vi "Catch.vi"(7 "Action":T1, 8 "error in (no error)":errorcluster) -> (0 "error out":errorcluster)   [LabVIEW 2015]
doc: "Wrapper for catching. It has the following actions:\n-PreCatch: sets the clapper to out, the roller pneumatic to in, actuates the kicker, and spins the roller motor forward.\n-Catch: sets the clapper to in.\n-Stop: deactuates the kicker, turns the roller motor off, and sets the roller pneumatic to middle."
uses:
  CatchAction.ctl
  DoubleSolenoidAction.ctl
  RollerAction.ctl
  SingleSolenoidAction.ctl
  PnuematicMode.ctl
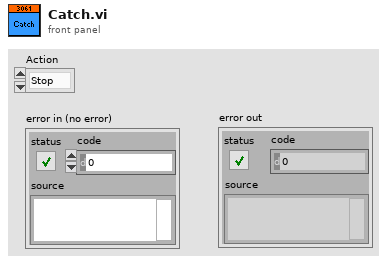
[diagram p1: front panel]
types:
  T1 = typedef "CatchAction.ctl" = enum16{"Stop", "PreCatch", "Catch"}
  T2 = typedef "SingleSolenoidAction.ctl" = enum16{"Init", "SetState", "Disable"}
  T3 = typedef "RollerAction.ctl" = enum16{"Init", "Off", "Forward", "Reverse"}
  T4 = typedef "DoubleSolenoidAction.ctl" = enum16{"Init", "Middle", "In", "Out"}
  T5 = typedef "PnuematicMode.ctl" = enum16{"Init", "SetState", "Disable"}
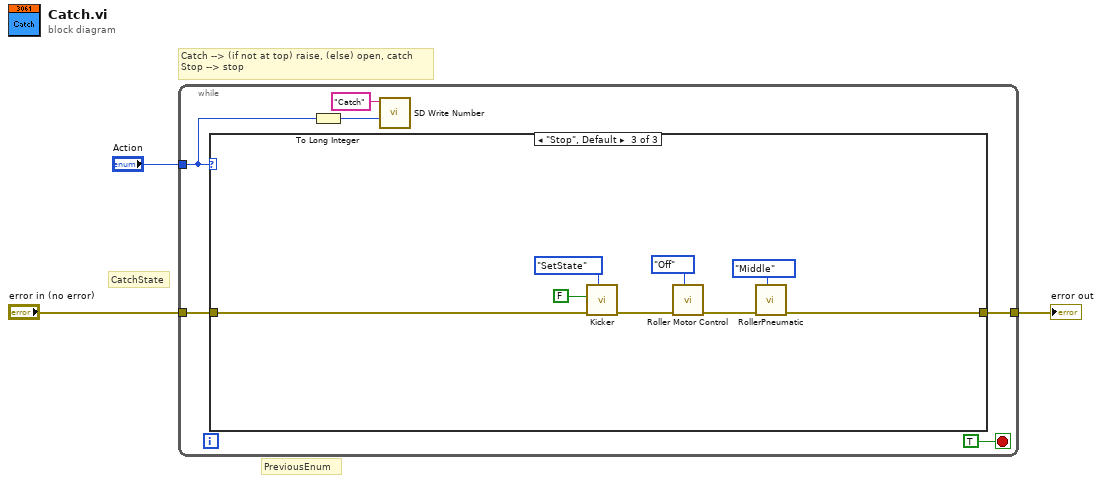
[diagram p0: block diagram]
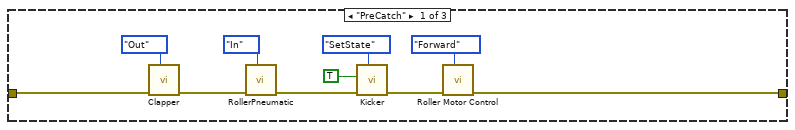
[diagram p2: hidden frame]
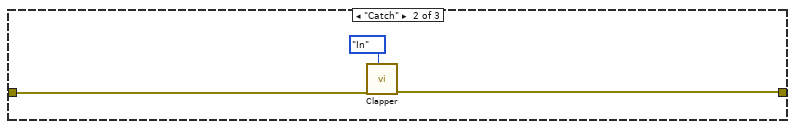
[diagram p3: hidden frame]
diagram:
  # "CatchState"
  # "Catch --> (if not at top) raise, (else) open, catch\nStop --> stop"
  # "PreviousEnum"
  n1 = while {
    tunnel: "error in (no error)" -> [w9]
    tunnel: [w8] -> w2
    tunnel: "Action" -> [w4]
    stop <- TRUE stop-if-true
    n2 = case shown="\"Stop\", Default" w4 {
      tunnel: w9 -> [w14 w21 w26]
      tunnel: [w12 w20 w24] -> w8
      frame "PreCatch" {
        n3 = call "Clapper.vi"("State"=DoubleSolenoidAction."Out", "Error in"=w14) -> ("Error out"=w15:errorcluster)  [unwired: 9 in]
        n4 = call "RollerPneumatic.vi"("State"=DoubleSolenoidAction."In", "Error in"=w15) -> ("Error out"=w16:errorcluster)  [unwired: 9 in]
        n5 = call "Kicker.vi"("Action"=SingleSolenoidAction."SetState", "error in (no error)"=w16, "Actuate?"=TRUE) -> ("error out"=w13:errorcluster)  [unwired: 8 in]
        n6 = call "Roller Motor Control.vi"("Action"=RollerAction."Forward", "Error in"=w13) -> ("Error out"=w12:errorcluster)  [unwired: 9 in]
      }
      frame "Catch" {
        n7 = call "Clapper.vi"("State"=DoubleSolenoidAction."In", "Error in"=w21) -> ("Error out"=w20:errorcluster)  [unwired: 9 in]
      }
      frame "Stop", Default {
        n8 = call "Kicker.vi"("Action"=PnuematicMode."SetState" ("Mode"), "error in (no error)"=w26, "Actuate?"=FALSE) -> ("error out"=w28:errorcluster)  [unwired: 8 in]
        n9 = call "Roller Motor Control.vi"("Action"=RollerAction."Off", "Error in"=w28) -> ("Error out"=w25:errorcluster)  [unwired: 9 in]
        n10 = call "RollerPneumatic.vi"("State"=DoubleSolenoidAction."Middle", "Error in"=w25) -> ("Error out"=w24:errorcluster)  [unwired: 9 in]
      }
    }
    n11 = To Long Integer(number=w4) -> (32bit integer=w6:i32)
    n12 = call <vilib>:"SD Write Number.vi"("Numeric"=w6, "Name"="Catch") -> ()  [unwired: 8 in, 2 out]
  }
  "error out" <- w2
